vi "alignRightWith.vi"(6 "useControlBodyOnly":bool, 8 "error in (no error)":errorcluster, 10 "anchorObject":refnum<vi>, 11 "movingObject":refnum<vi>) -> (0 "error out":errorcluster, 2 "anchorObject(dup)":refnum<vi>, 3 "movingObject(dup)":refnum<vi>)   [LabVIEW 2023]
doc: "Align right the 'movingObject' with the 'anchorObject'.\n\nOnly the X position of the item is modified.\nThe Y position is preserved."
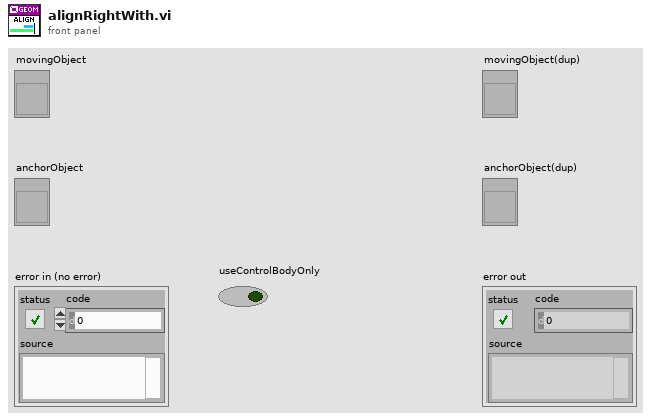
[diagram p1: front panel]
types:
  T1 = cluster{"left":i32, "top":i32, "right":i32, "bottom":i32}
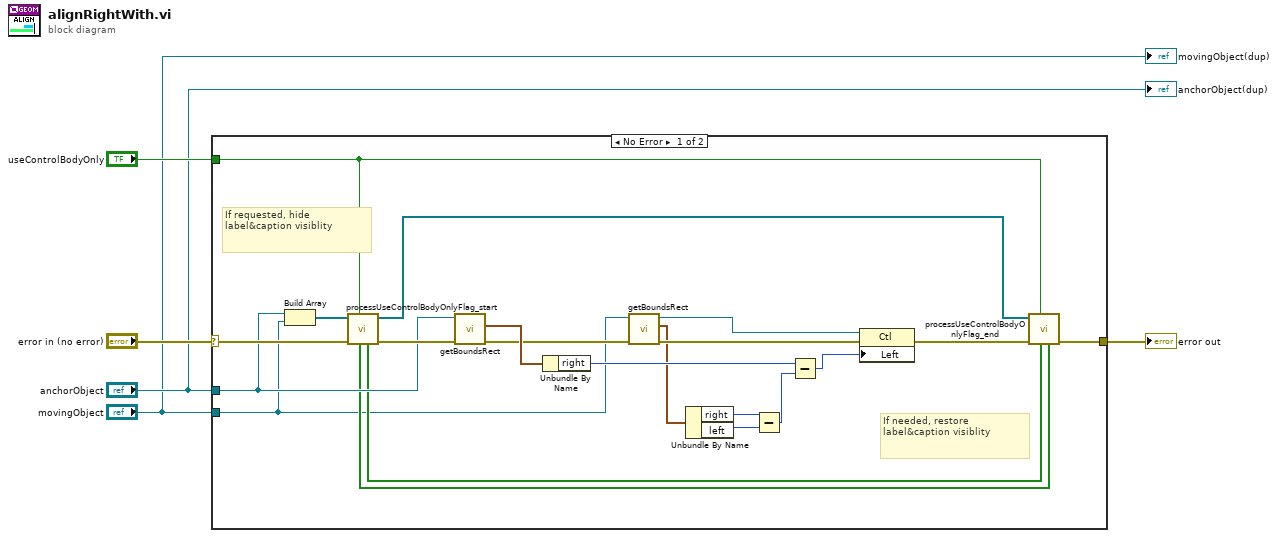
[diagram p0: block diagram]
diagram:
  n1 = case shown="No Error" "error in (no error)" {
    selector: "error in (no error)" -> [w26 w27]
    tunnel: [w23 w27] -> w5
    tunnel: "anchorObject" -> [w21 _]
    tunnel: "useControlBodyOnly" -> [w18 _]
    tunnel: "movingObject" -> [w11 _]
    frame No Error {
      # "If needed, restore label&caption visiblity"
      # "If requested, hide label&caption visiblity"
      n2 = Build Array(w21, w11) -> (w25:refnum<vi>[])
      n3 = call "processUseControlBodyOnlyFlag_start.vi"("useControlBodyOnly"=w18, "error in (no error)"=w26, "refList"=w25) -> ("error out"=w22:errorcluster, "refList(dup)"=w24:refnum<vi>[], "LabelVisibilityList"=w17:bool[], "captionVisibilityList"=w16:bool[])  [unwired: 5 in]
      n4 = call "getBoundsRect.vi"("error in (no error)"=w22, "ref"=w21) -> ("error out"=w14:errorcluster, "rect"=w20:T1)  [unwired: 7 in, 1 out]
      n5 = Unbundle By Name(w20) -> ("right"=w15:i32)
      n6 = call "getBoundsRect.vi"("error in (no error)"=w14, "ref"=w11) -> ("error out"=w13:errorcluster, "rect"=w10:T1, "ref(dup)"=w12:refnum<vi>)  [unwired: 7 in]
      n7 = Unbundle By Name(w10) -> ("right"=w9:i32, "left"=w8:i32)
      n8 = Subtract(x=w9, y=w8) -> (x-y=w6:i32)
      n9 = Subtract(x=w15, y=w6) -> (x-y=w7:i32)
      n10 = property class="Ctl"(reference=w12, error in=w13, "Left"=w7) -> (error out=w19:errorcluster)  [unwired: 1 out]
      n11 = call "processUseControlBodyOnlyFlag_end.vi"("captionVisibilityList"=w16, "LabelVisibilityList"=w17, "useControlBodyOnly"=w18, "error in (no error)"=w19, "refList"=w24) -> ("error out"=w23:errorcluster)  [unwired: 5 in, 1 out]
    }
    frame Error {
    }
  }
  "error out" <- w5
  "movingObject(dup)" <- "movingObject"
  "anchorObject(dup)" <- "anchorObject"
